vi "Grenzwerte aendern.vi"(6 "Auswahl":enum16{"Min", "Max"}(ring), 9 "Grenzen Max":T1 {"Zahlen-Eingabefeld 16" format="%#_5g"; "Zahlen-Eingabefeld 15" format="%#_5g"; "Zahlen-Eingabefeld 14" format="%#_5g"; "Zahlen-Eingabefeld 13" format="%#_5g"; "Zahlen-Eingabefeld 12" format="%#_5g"; "Zahlen-Eingabefeld 11" format="%#_5g"; "Zahlen-Eingabefeld 10" format="%#_5g"; "Zahlen-Eingabefeld 9" format="%#_5g"; "Zahlen-Eingabefeld 8" format="%#_5g"; "Zahlen-Eingabefeld 7" format="%#_5g"; "Zahlen-Eingabefeld 6" format="%#_5g"; "Zahlen-Eingabefeld 5" format="%#_5g"; "Zahlen-Eingabefeld 4" format="%#_5g"; "Zahlen-Eingabefeld 3" format="%#_5g"; "Zahlen-Eingabefeld 2" format="%#_5g"; "Zahlen-Eingabefeld" format="%#_5g"}, 10 "Grenzen Min":T1 {"Zahlen-Eingabefeld 16" format="%#_5g"; "Zahlen-Eingabefeld 15" format="%#_5g"; "Zahlen-Eingabefeld 14" format="%#_5g"; "Zahlen-Eingabefeld 13" format="%#_5g"; "Zahlen-Eingabefeld 12" format="%#_5g"; "Zahlen-Eingabefeld 11" format="%#_5g"; "Zahlen-Eingabefeld 10" format="%#_5g"; "Zahlen-Eingabefeld 9" format="%#_5g"; "Zahlen-Eingabefeld 8" format="%#_5g"; "Zahlen-Eingabefeld 7" format="%#_5g"; "Zahlen-Eingabefeld 6" format="%#_5g"; "Zahlen-Eingabefeld 5" format="%#_5g"; "Zahlen-Eingabefeld 4" format="%#_5g"; "Zahlen-Eingabefeld 3" format="%#_5g"; "Zahlen-Eingabefeld 2" format="%#_5g"; "Zahlen-Eingabefeld" format="%#_5g"}, 11 "Ref Auswahlfelder":refnum<vi>[](array[refnum])) -> ()   [LabVIEW 2020, in "Gaszuordnung AO.lvlib"]
uses:
  Gaszuordnung AO.lvlib
  Grenzen Anzeige.ctl
  Visualisierungs Elemente/Zahlen-Eingabefeld.ctl
  FGV Gaszuordnung Grenzen&Einheit Aktion.ctl
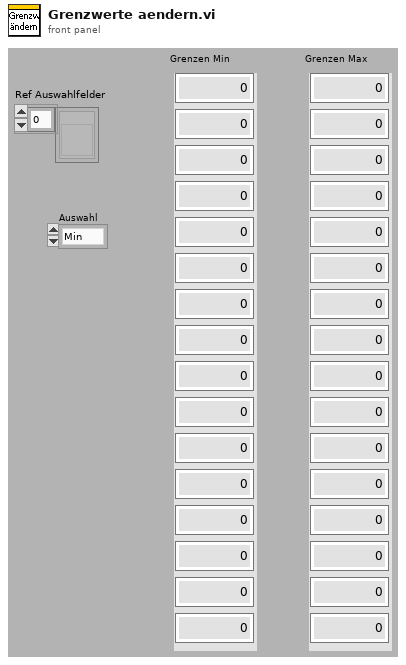
[diagram p1: front panel]
types:
  T1 = typedef "Gaszuordnung AO.lvlib/Grenzen Anzeige.ctl" = cluster{"Zahlen-Eingabefeld":T2, "Zahlen-Eingabefeld 2":T2, "Zahlen-Eingabefeld 3":T2, "Zahlen-Eingabefeld 4":T2, "Zahlen-Eingabefeld 5":T2, "Zahlen-Eingabefeld 6":T2, "Zahlen-Eingabefeld 7":T2, "Zahlen-Eingabefeld 8":T2, "Zahlen-Eingabefeld 9":T2, "Zahlen-Eingabefeld 10":T2, "Zahlen-Eingabefeld 11":T2, "Zahlen-Eingabefeld 12":T2, "Zahlen-Eingabefeld 13":T2, "Zahlen-Eingabefeld 14":T2, "Zahlen-Eingabefeld 15":T2, "Zahlen-Eingabefeld 16":T2}
  T2 = typedef "Zahlen-Eingabefeld.ctl" = sgl
  T3 = typedef "Gaszuordnung AO.lvlib/FGV Gaszuordnung Grenzen&Einheit Aktion.ctl" = enum16{"Lesen", "Schreiben Min", "Schreiben Max", "Laden", "Speichern"}
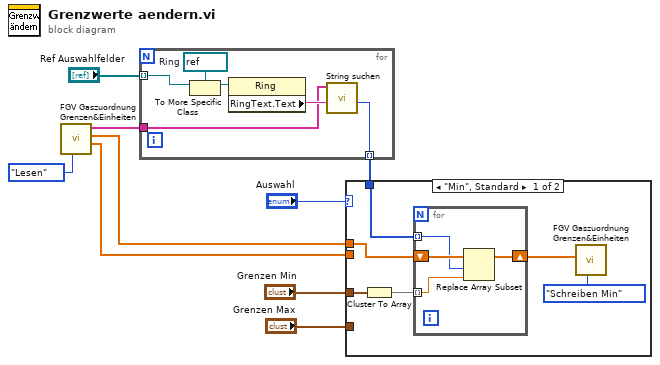
[diagram p0: block diagram]
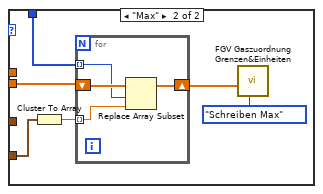
[diagram p2: hidden frame]
diagram:
  n1 = call "FGV Gaszuordnung Grenzen&Einheiten.vi"("Aktion"=FGV_Gaszuordnung_Grenzen&Einheit_Aktion."Lesen") -> ("Max neu"=w5:dbl[], "Min neu"=w1:dbl[], "Namen neu"=w8:string[])  [unwired: 2 in, 6 out]
  n2 = for {
    tunnel: "Ref Auswahlfelder" -> [w14] mode=indexing
    tunnel: w8 -> [w10]
    tunnel: [w12] -> w4 mode=indexing
    w15 = refnum<vi> refnum  # Ring
    n3 = To More Specific Class(target class=w15, reference=w14) -> (specific class reference=w13:refnum<vi>)  [unwired: 1 in, 1 out]
    n4 = property class="Ring"(reference=w13) -> ("RingText.Text"=w11:string)  [unwired: 1 in, 2 out]
    n5 = call "String suchen.vi"("Gasname"=w11, "Such-Namen"=w10) -> ("Index"=w12:i32)  [unwired: 8 in, 1 out]
  }
  n6 = case shown="\"Min\", Standard" "Auswahl" {
    tunnel: w5 -> [_ w30]
    tunnel: w4 -> [w19 w29]
    tunnel: "Grenzen Max" -> [_ w28]
    tunnel: "Grenzen Min" -> [w18 _]
    tunnel: w1 -> [w17 _]
    frame "Min", Default {
      n7 = Cluster To Array(cluster=w18) -> (array=w21:T2[])
      n8 = for {
        shift-right: [w22] -> w16
        shift-left: w17 -> [w25]
        tunnel: w21 -> [w24] mode=indexing
        tunnel: w19 -> [w23] mode=indexing
        n9 = Replace Array Subset(array=w25, new element=w24, index=w23) -> (w22:dbl[])
      }
      n10 = call "FGV Gaszuordnung Grenzen&Einheiten.vi"("Aktion"=FGV_Gaszuordnung_Grenzen&Einheit_Aktion."Schreiben Min", "Min"=w16) -> ()  [unwired: 1 in, 9 out]
    }
    frame "Max" {
      n11 = Cluster To Array(cluster=w28) -> (array=w31:T2[])
      n12 = for {
        shift-right: [w32] -> w26
        shift-left: w30 -> [w35]
        tunnel: w31 -> [w34] mode=indexing
        tunnel: w29 -> [w33] mode=indexing
        n13 = Replace Array Subset(array=w35, new element=w34, index=w33) -> (w32:dbl[])
      }
      n14 = call "FGV Gaszuordnung Grenzen&Einheiten.vi"("Aktion"=FGV_Gaszuordnung_Grenzen&Einheit_Aktion."Schreiben Max", "Max"=w26) -> ()  [unwired: 1 in, 9 out]
    }
  }
